vi "Update Card Count.vi"(8 "new element/subarray":bool, 9 "Card Array in":bool[](array[boolean]), 10 "# in":u32, 11 "Message Enqueuer":refnum<class "Message Enqueuer.lvclass">) -> (1 "Card Array Out":bool[](array[boolean]), 3 "Message Enqueuer out":refnum<class "Message Enqueuer.lvclass">)   [LabVIEW 2012, in "Universal Power Meter.lvlib" / "Universal Power Meter.lvclass"]
uses:
  Universal Power Meter.lvclass
  <vilib>/ActorFramework/Message Enqueuer/Message Enqueuer.lvclass
  Universal Power Meter Messages/Write Card Array Msg/Write Card Array Msg.lvclass/Write Card Array Msg.ctl
  <vilib>/ActorFramework/Message Enqueuer/Message Enqueuer.lvclass/Message Enqueuer.ctl
  <vilib>/ActorFramework/Message Enqueuer/Enqueue.vi
  <vilib>/ActorFramework/Message Priority Queue/Priority Enqueue.vi
  Universal Power Meter Messages/Write Card Array Msg/Write Card Array Msg.lvclass
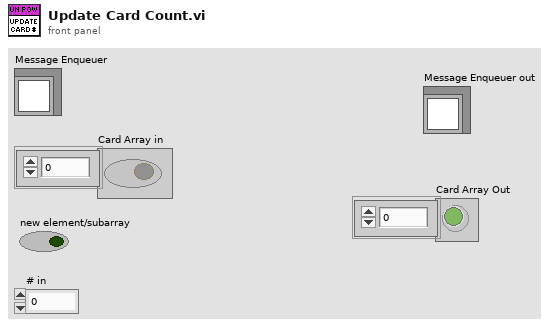
[diagram p1: front panel]
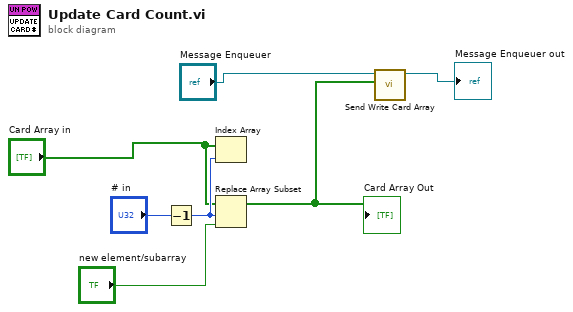
[diagram p0: block diagram]
diagram:
  n1 = Decrement(x="# in") -> (x-1=w6:u32)
  n2 = Index Array(array="Card Array in", index=w6) -> ()  [unwired: 1 out]
  n3 = Replace Array Subset(array="Card Array in", new element="new element/subarray", index=w6) -> (w3:bool[])
  "Card Array Out" <- w3
  n4 = call "Send Write Card Array.vi"("Value"=w3, "Message Enqueuer"="Message Enqueuer") -> ("Message Enqueuer out"=→"Message Enqueuer out":refnum<class "Message Enqueuer.lvclass">)  [unwired: 8 in, 1 out]
